vi "SFP Format Device Info for Table.vi"(11 "values":T1 {"Device Info"."Serial Number" format="%x"}) -> (3 "Info Table":string[][](table))   [LabVIEW 2017]
uses:
  <vilib>/addons/Sound and Vibration/svt_DAQmx/subVIs/SFP DAQmx Device Info.ctl
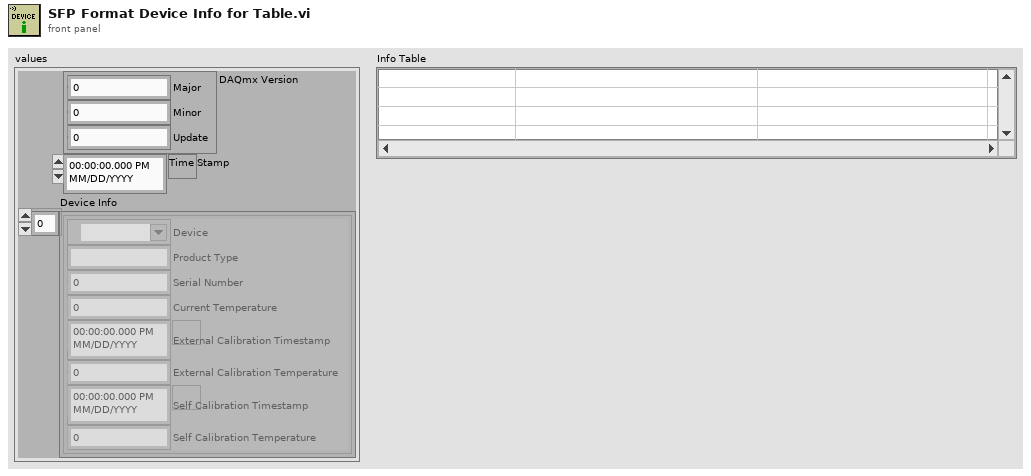
[diagram p1: front panel]
types:
  T1 = typedef "SFP DAQmx Device Info.ctl" = cluster{"DAQmx Version":cluster{"Major":u32, "Minor":u32, "Update":u32}, "Time Stamp":timestamp, "Device Info":cluster{"Device":tag, "Product Type":string, "Serial Number":u32, "Current Temperature":dbl, "External Calibration Timestamp":timestamp, "External Calibration Temperature":dbl, "Self Calibration Timestamp":timestamp, "Self Calibration Temperature":dbl}[]}
  T2 = cluster{"Device":tag, "Product Type":string, "Serial Number":u32, "Current Temperature":dbl, "External Calibration Timestamp":timestamp, "External Calibration Temperature":dbl, "Self Calibration Timestamp":timestamp, "Self Calibration Temperature":dbl}[]
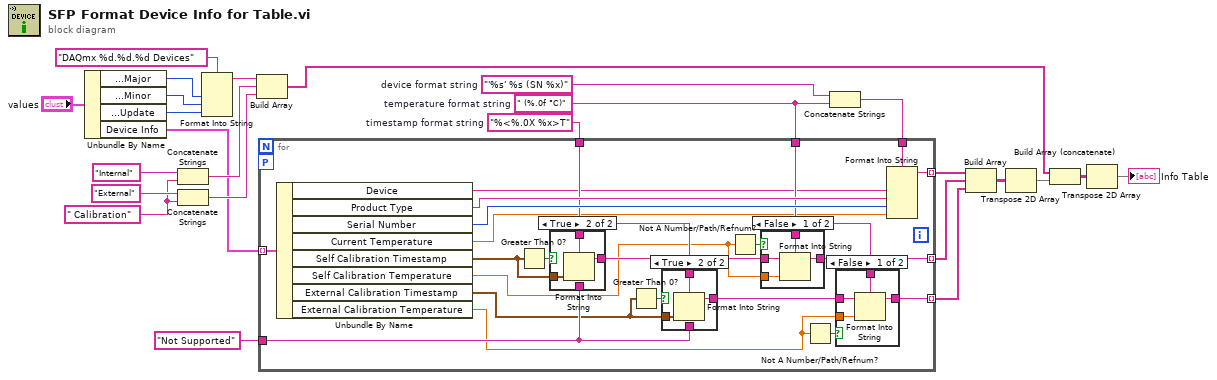
[diagram p0: block diagram]
diagram:
  w10 = " (%.0f °C)"  # temperature format string
  w23 = "%<%.0X %x>T"  # timestamp format string
  w9 = "'%s' %s (SN %x)"  # device format string
  w16 = " Calibration" ("initial string")
  n1 = Unbundle By Name("values") -> ("DAQmx Version.Major"=w12:u32, "DAQmx Version.Minor"=w13:u32, "DAQmx Version.Update"=w14:u32, "Device Info"=w2:T2)
  n2 = Concatenate Strings("Internal" ("initial string"), w16) -> (w20:string)
  n3 = Concatenate Strings("External" ("initial string"), w16) -> (w21:string)
  n4 = Format Into String(format string="DAQmx %d.%d.%d Devices", w12, w13, w14) -> (resulting string=w19:string)  [unwired: 2 in, 1 out]
  n5 = Build Array(w19, w20, w21) -> (w1:string[])
  n6 = Concatenate Strings(w9, w10) -> (w8:string)
  n7 = for {
    tunnel: w2 -> [w45] mode=indexing
    tunnel: [w44] -> w7 mode=indexing
    tunnel: [w43] -> w6 mode=indexing
    tunnel: [w37] -> w5 mode=indexing
    tunnel: w8 -> [w42]
    tunnel: w23 -> [w41]
    tunnel: w10 -> [w40]
    tunnel: "Not Supported" ("format string") -> [w31]
    workers-P: _ -> [_]
    n8 = Unbundle By Name(w45) -> ("Device"=w29:tag, "Product Type"=w47:string, "Serial Number"=w46:u32, "Current Temperature"=w30:dbl, "Self Calibration Timestamp"=w32:timestamp, "Self Calibration Temperature"=w26:dbl, "External Calibration Timestamp"=w27:timestamp, "External Calibration Temperature"=w28:dbl)
    n9 = Greater Than 0?(x=w32) -> (x > 0?=w33:bool)
    n10 = case shown="True" w33 {
      tunnel: w32 -> [_ w51]
      tunnel: w41 -> [_ w50]
      tunnel: [w48 w49] -> w39
      tunnel: w31 -> [w48 _]
      frame False {
      }
      frame True {
        n11 = Format Into String(format string=w50, w51) -> (resulting string=w49:string)  [unwired: 2 in, 1 out]
      }
    }
    n12 = Greater Than 0?(x=w27) -> (x > 0?=w34:bool)
    n13 = case shown="True" w34 {
      tunnel: w41 -> [_ w55]
      tunnel: [w52 w54] -> w38
      tunnel: w27 -> [_ w53]
      tunnel: w31 -> [w52 _]
      frame False {
      }
      frame True {
        n14 = Format Into String(format string=w55, w53) -> (resulting string=w54:string)  [unwired: 2 in, 1 out]
      }
    }
    n15 = Not A Number/Path/Refnum?(number/path/refnum=w26) -> (NaN/Path/Refnum?=w36:bool)
    n16 = case shown="False" w36 {
      tunnel: w26 -> [w64 _]
      tunnel: [w63 w65] -> w43
      tunnel: w40 -> [w62 _]
      tunnel: w39 -> [w61 w65]
      frame False {
        n17 = Format Into String(format string=w62, initial string=w61, w64) -> (resulting string=w63:string)  [unwired: 1 in, 1 out]
      }
      frame True {
      }
    }
    n18 = Not A Number/Path/Refnum?(number/path/refnum=w28) -> (NaN/Path/Refnum?=w35:bool)
    n19 = case shown="False" w35 {
      tunnel: w28 -> [w59 _]
      tunnel: w40 -> [w58 _]
      tunnel: w38 -> [w57 w60]
      tunnel: [w56 w60] -> w37
      frame False {
        n20 = Format Into String(format string=w58, initial string=w57, w59) -> (resulting string=w56:string)  [unwired: 1 in, 1 out]
      }
      frame True {
      }
    }
    n21 = Format Into String(format string=w42, w29, w47, w46, w30) -> (resulting string=w44:string)  [unwired: 2 in, 1 out]
  }
  n22 = Build Array(w7, w6, w5) -> (w4:string[][])
  n23 = Transpose 2D Array(2D array=w4) -> (transposed array=w3:string[][])
  n24 = Build Array (concatenate)(w1, w3) -> (w22:string[][])
  n25 = Transpose 2D Array(2D array=w22) -> (transposed array=→"Info Table":string[][])
